vi "CANFD_SizetoIndex.vi"(11 "Payload Size":i32) -> (3 "Duration Index":i32)   [LabVIEW 2019, in "XNET-Bus-Load-Calculator.lvlib" / "CANBus_Load_Calculator.lvclass"]
uses:
  CANBus_Load_Calculator.lvclass
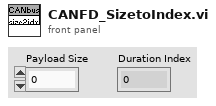
[diagram p1: front panel]
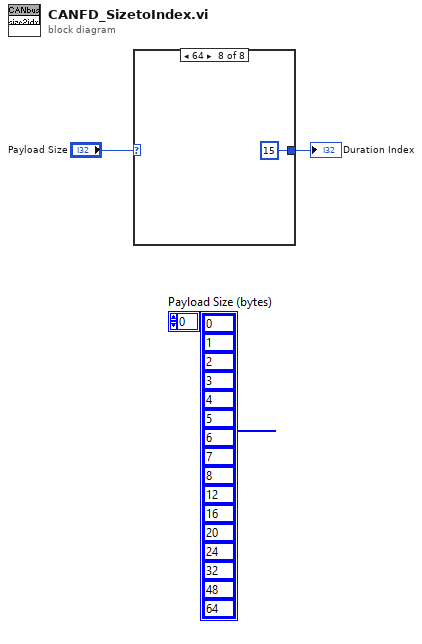
[diagram p0: block diagram]
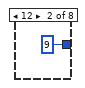
[diagram p3: hidden frame]
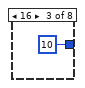
[diagram p4: hidden frame]
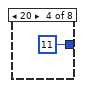
[diagram p5: hidden frame]
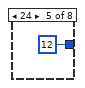
[diagram p6: hidden frame]
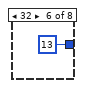
[diagram p7: hidden frame]
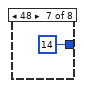
[diagram p8: hidden frame]
diagram:
  n1 = case shown="64" "Payload Size" {
    selector: "Payload Size" -> [w3 _ _ _ _ _ _ _]
    tunnel: [w3 9 ("Payload Size") 10 ("Payload Size") 11 ("Payload Size") 12 ("Payload Size") 13 ("Payload Size") 14 ("Payload Size") 15 ("Payload Size")] -> w1
    frame Default {
    }
    frame 12 {
    }
    frame 16 {
    }
    frame 20 {
    }
    frame 24 {
    }
    frame 32 {
    }
    frame 48 {
    }
    frame 64 {
    }
  }
  "Duration Index" <- w1
